vi "RobotDrive.vi"(11 "Drive":cluster{"RobotDriveDevRef":T1}) -> ()   [LabVIEW 2014]
uses:
  <vilib>/Rock Robotics/WPI/RobotDrive/WPI_RobotDriveDevRef.ctl
  <vilib>/Rock Robotics/WPI/MotorControl/WPI_MotorControlDeviceRef.ctl
  <vilib>/Rock Robotics/WPI/MotorControl/WPI_MotorControlType.ctl
  <vilib>/Rock Robotics/SystemInterfaces/Typedef/FPGA_TypedefDigitalModule.ctl
  <vilib>/Rock Robotics/SystemInterfaces/DIO/FPGA_DIOPWMChannel.ctl
  <vilib>/Rock Robotics/WPI/PWM/WPI_PWMDeadband.ctl
  <vilib>/Rock Robotics/WPI/CAN/Jaguar/SubVIs/WPI_CANJaguar_ControlMode.ctl
  <vilib>/Rock Robotics/WPI/CAN/TalonSRX/WPI_CANTalonSRX_APIControlMode.ctl
  <vilib>/Rock Robotics/WPI/PWM/WPI_PWMTransform_ConPane.ctl
  Robot Values.vi
  DriveGlobal.vi
  Robot Fail.vi
  <vilib>/ptbypt/NI_PtbyPt.lvlib
panel:
  in  "Left Scale factor":dbl=0.7 format="%#_13g"
  in  "Right scale factor":dbl=0.8 format="%#_13g"
  in  "Filter on":bool=TRUE
  in  "low cutoff freq: fl":dbl=0.9999999999999999 format="%0.3f"
  in  "order":i32=1
  in  "sampling freq: fs":dbl=50.0 format="%0.2f"
  in  "initialize":bool
  # "Values for filtering the desired motor values from \nRobot Values.vi global. They arejust approximations\nand will need to be tuned for the drivers."
  # "Press this to update the values\ndurring testing, or restart the code"
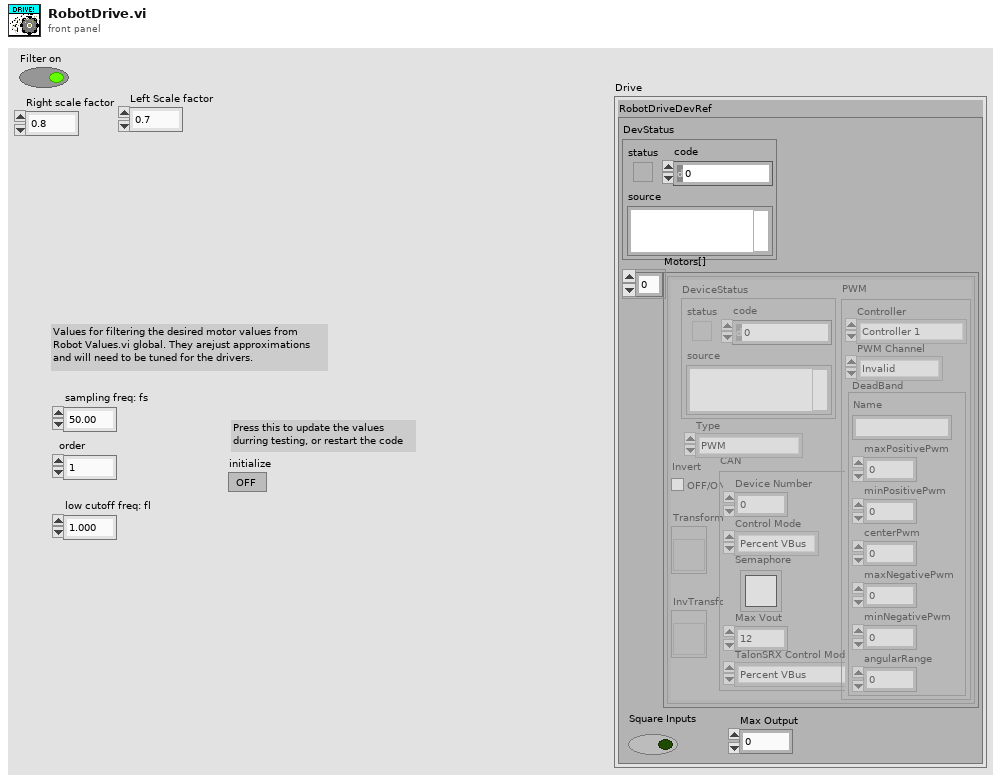
[diagram p1: front panel]
types:
  T1 = typedef "WPI_RobotDriveDevRef.ctl" = cluster{"DevStatus":errorcluster, "Motors[]":T2[], "Square Inputs":bool, "Max Output":dbl}
  T2 = typedef "WPI_MotorControlDeviceRef.ctl" = cluster{"DeviceStatus":errorcluster, "Type":T3, "PWM":cluster{"Controller":T4, "PWM Channel":T5, "DeadBand":T6}, "CAN":cluster{"Device Number":u8, "Control Mode":T7, "Semaphore":T8, "Max Vout":dbl, "TalonSRX Control Mode":T9}, "Invert":bool, "TransformRef":T10, "InvTransformRef":T10}
  T3 = typedef "WPI_MotorControlType.ctl" = enum16{"PWM", "CAN", "CANTalonSRX"}
  T4 = typedef "FPGA_TypedefDigitalModule.ctl" = enum16{"Controller 1"}
  T5 = typedef "FPGA_DIOPWMChannel.ctl" = enum8{"PWM 0", "PWM 1", "PWM 2", "PWM 3", "PWM 4", "PWM 5", "PWM 6", "PWM 7", "PWM 8", "PWM 9", "PWM MXP 0", "PWM MXP 1", "PWM MXP 2", "PWM MXP 3", "PWM MXP 4", "PWM MXP 5", "PWM MXP 6", "PWM MXP 7", "PWM MXP 8", "PWM MXP 9", "Invalid"}
  T6 = typedef "WPI_PWMDeadband.ctl" = cluster{"Name":string, "maxPositivePwm":i32, "minPositivePwm":i32, "centerPwm":i32, "maxNegativePwm":i32, "minNegativePwm":i32, "angularRange":u16}
  T7 = typedef "WPI_CANJaguar_ControlMode.ctl" = enum8{"Percent VBus", "Current", "Speed", "Position", "Voltage"}
  T8 = typedef "Semaphore RefNum" = refnum<k1>
  T9 = typedef "WPI_CANTalonSRX_APIControlMode.ctl" = enum8{"Percent VBus", "Speed", "Position", "Slave", "Unchanged / Invalid"}
  T10 = typedef "WPI_PWMTransform_ConPane.ctl" = refnum<vi>
  T11 = cluster{"RightMotorSpeed":dbl, "LeftMotorSpeed":dbl}
  T12 = cluster{"Tracking Tote?":bool, "ToteRightSpeed":dbl, "ToteLeftSpeed":dbl, "Drive Encoder reset":bool, "Right Wheel \n(Cm)":dbl, "Left Wheel \n(Cm)":dbl}
  T13 = cluster{"Not stright - Right":bool, "Not stright - Left":bool, "Lift position change":bool, "Lift out of sync":bool, "Joystick sensitivity Less":bool, "Stuck in Tank":bool, "Joystick Sensistiviy More":bool}
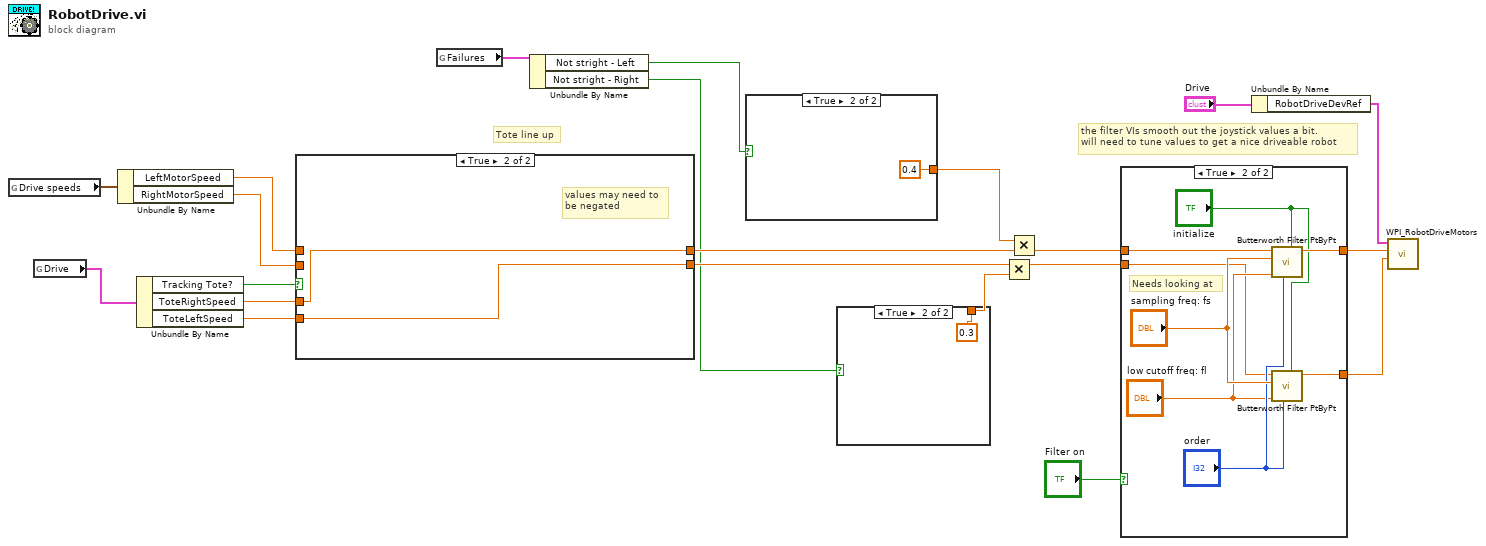
[diagram p0: block diagram]
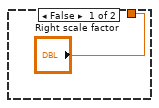
[diagram p2: hidden frame]
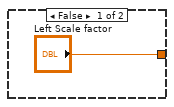
[diagram p3: hidden frame]
diagram:
  # "Tote line up"
  # "the filter VIs smooth out the joystick values a bit.\nwill need to tune values to get a nice driveable robot"
  n1 = global read "DriveGlobal.vi" "Drive speeds"() -> (w10:T11)
  n2 = global read "Robot Values.vi" "Drive"() -> (w19:T12)
  n3 = Unbundle By Name(w10) -> ("LeftMotorSpeed"=w9:dbl, "RightMotorSpeed"=w8:dbl)
  n4 = Unbundle By Name(w19) -> ("Tracking Tote?"=w14:bool, "ToteRightSpeed"=w13:dbl, "ToteLeftSpeed"=w12:dbl)
  n5 = case shown="True" w14 {
    tunnel: [w23 w25] -> w16
    tunnel: w9 -> [w23 _]
    tunnel: [w22 w24] -> w15
    tunnel: w8 -> [w22 _]
    tunnel: w13 -> [_ w25]
    tunnel: w12 -> [_ w24]
    frame False {
      # "Do nothing, we're not\ntracking the tote\nso no eidts need to \nbe made to values"
    }
    frame True {
      # "values may need to\nbe negated"
    }
  }
  n6 = global read "Robot Fail.vi" "Failures"() -> (w3:T13)
  n7 = Unbundle By Name(w3) -> ("Not stright - Left"=w2:bool, "Not stright - Right"=w1:bool)
  n8 = case shown="True" w2 {
    tunnel: ["Left Scale factor" 0.4 ("Left Scale factor")] -> w6
    frame False {
    }
    frame True {
    }
  }
  n9 = case shown="True" w1 {
    tunnel: ["Right scale factor" 0.3 ("Right scale factor")] -> w4
    frame False {
    }
    frame True {
    }
  }
  n10 = Multiply(x=w15, y=w4) -> (x*y=w5:dbl)
  n11 = Multiply(x=w6, y=w16) -> (x*y=w7:dbl)
  n12 = case shown="True" "Filter on" {
    tunnel: [w31 w39] -> w18
    tunnel: [w30 w38] -> w17
    tunnel: w7 -> [w31 w33]
    tunnel: w5 -> [w30 w32]
    frame False {
    }
    frame True {
      # "Needs looking at"
      n13 = call <vilib>:"Butterworth Filter PtByPt.vi"("initialize"="initialize", "order"="order", "low cutoff freq: fl"="low cutoff freq: fl", "sampling freq: fs"="sampling freq: fs", "x"=w33) -> ("Filtered x"=w39:dbl)  [unwired: 4 in, 1 out]
      n14 = call <vilib>:"Butterworth Filter PtByPt.vi"("initialize"="initialize", "order"="order", "low cutoff freq: fl"="low cutoff freq: fl", "sampling freq: fs"="sampling freq: fs", "x"=w32) -> ("Filtered x"=w38:dbl)  [unwired: 4 in, 1 out]
    }
  }
  n15 = Unbundle By Name("Drive") -> ("RobotDriveDevRef"=w20:T1)
  n16 = call <vilib>:"WPI_RobotDriveMotors.vi"("RightSpeed"=w17, "LeftSpeed"=w18, "RobotDriveDevRef"=w20) -> ()  [unwired: 6 in, 3 out]
